vi "Clear Chassis Tasks.vi"(8 "error in (no error)":errorcluster, 11 "Chassis Tasks in":refnum<class "Chassis Tasks.lvclass">) -> (0 "error out":errorcluster, 3 "Chassis Tasks out":refnum<class "Chassis Tasks.lvclass">)   [LabVIEW 2012, in "Data Acquisition.lvlib" / "Chassis Tasks.lvclass"]
uses:
  Chassis Tasks.lvclass
  Chassis Tasks.lvclass/Chassis Tasks.ctl
  Class DAQ Task/DAQ Task.lvclass
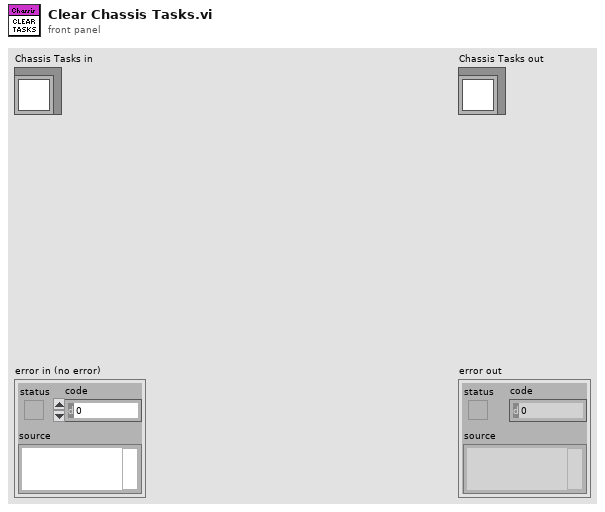
[diagram p1: front panel]
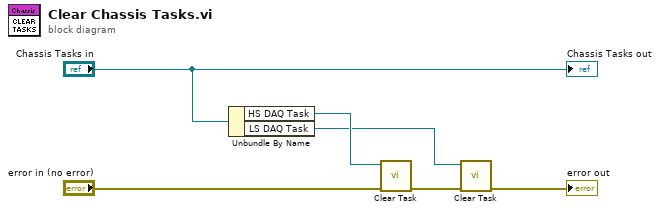
[diagram p0: block diagram]
diagram:
  n1 = Unbundle By Name("Chassis Tasks in") -> ("HS DAQ Task"=w2:refnum<class "DAQ Task.lvclass">, "LS DAQ Task"=w1:refnum<class "DAQ Task.lvclass">)
  n2 = call "Clear Task.vi"("error in (no error)"="error in (no error)", "DAQ Task in"=w2) -> ("error out"=w3:errorcluster)  [unwired: 8 in, 1 out]
  n3 = call "Clear Task.vi"("error in (no error)"=w3, "DAQ Task in"=w1) -> ("error out"=→"error out":errorcluster)  [unwired: 8 in, 1 out]
  "Chassis Tasks out" <- "Chassis Tasks in"
